vi "DARPA_DoubleJ_20220815_Arduino_ver_newpump.vi"() -> ()   [LabVIEW 2021]
uses:
  <vilib>/Instr/_visa.llb/VISA Configure Serial Port (Instr).vi
  <vilib>/FPGAPlugInAG/PCIe-7857/niLvFpga_Open_PCIe-7857.vi
  <vilib>/rvi/interface/common/dynamic/niFpgaDynamicAddResources.vi
  <vilib>/Utility/error.llb/Error Cluster From Error Code.vi
  <vilib>/rvi/errors/niLvFpgaAdjustHostInterfaceError.vi
  <vilib>/FPGAPlugInAG/Dynamic/niLvFpga_Close_Dynamic.vi
  <vilib>/rvi/interface/nirviOpenFPGA/nirviOpenFPGA.xnode
  FPGA Bitfiles/darpatransitionj_FPGATarget_DARPAFPGADoubleJ_E+A750Kw4Ow.lvbitx
  DARPA_FPGA_DoubleJ_20220715.vi
  <vilib>/rvi/interface/nirviReadWriteControl/nirviReadWriteControl.xnode
  <vilib>/rvi/interface/nirviCloseFPGA/nirviCloseFPGA.xnode
  NiFpgaLv.dll
  <vilib>/rvi/interface/Simulation/niFpgaSimulationCallBeginRW.vi
  <instrlib>/KD Scientific Legato 2XX Series/KD Scientific Legato 2XX Series.lvlib
panel:
  out "Diameter1 (mm)":dbl=4.699
  in  "dia1 (mm)":dbl=0.1 caption="Set Diameter (mm)" min=0.1 max=50.0
  in  "Syringe Selection1":string(combo)="BDP1MM"
  in  "Flow Rate Units (1:ml/min) 2":u32(ring)=1 items=["milliliters per hour (ml/hr)", "milliliters per minute (ml/min)", "milliliters per second (ml/sec)", "microliters per hour (ul/hr)", "microliters per minute (ul/min)", "microliters per second (ul/sec)", "nanoliters per hour (nl/hr)", "nanoliters per minute (nl/min)", "nanoliters per second (nl/sec)", "picoliters per hour (pl/hr)", "picoliters per minute (pl/min)", "picoliters per second (pl/sec)"]
  in  "Flow Rate (5) 2":dbl=5.0 format="%#.4f"
  in  "set param 1":bool
  in  "Baud Rate (115200)":u32(ring)=115200 items=["9600"=9600, "19200"=19200, "38400"=38400, "57600"=57600, "115200"=115200]
  in  "Infuse":bool
  in  "Pause":bool
  in  "Withdraw":bool
  in  "Stop":bool
  out "Infusing":bool
  out "Withdrawing":bool
  out "Idle":bool
  out "Infused Volume":dbl
  out "Withdrawn Volume":dbl
  out "Units (infused)":u16(ring) items=["milliliters", "microliters", "nanoliters", "picoliters"]
  out "Units (withdrawn)":u16(ring) items=["milliliters", "microliters", "nanoliters", "picoliters"]
  in  "VISA resource name":refnum<visa-resource-name>
  out "error out":errorcluster
  in  "stop":bool
  out "Image":u16[][](graph)
  in  "Display":bool=TRUE
  out "Total Frames":i32
  out "Elapsed Time":u32
  out "Software FPS":dbl
  out "Camera FPS":dbl
  in  "H Offset":i32 min=0 max=1604 step=4
  in  "H Width":i32 min=4 max=2304 step=4
  out "SMD":dbl
  out "SHO":i32
  in  "V Offset":i32 min=0 max=1604 step=4
  in  "V Width":i32 min=4 max=2304 step=4
  in  "Binning":u16(ring)=1 items=["1x1"=1, "2x2"=2, "4x4"=4]
  out "SHW":i32
  out "SVO":i32
  out "SVW":i32
  in  "Scan Mode":dbl min=1.0 max=3.0 step=1.0
  in  "Exposure":dbl min=6.576470588235294e-05 max=10.000017235294118 step=1e-08
  out "EXP":dbl
  out "Camera Model":string
  out "Camera Version":string
  out "Camera Serial":string
  in  "Merger on":bool
  in  "ratiocontrol":dbl=1.0
  in  "Arduino COM port":refnum<visa-resource-name>="COM10"
  in  "Arduino \nshut down":bool=TRUE
  in  "Initializer":bool
  out "Serial debugger":string
  in  "PMT2 senstivity":bool
  in  "PMT1 senstivity":bool
  in  "Func amp":bool
  in  "Func Freq":bool
  in  "Func On time":bool
  in  "Func Delay":bool
  in  "PMT1 senstivity input":dbl=0.7 caption="0.5-0.75 V"
  in  "PMT2 senstivity input":dbl caption="0.5-0.75 V"
  in  "Func amp input":dbl=5.0 caption="0 - 5 V"
  in  "Func freq input":dbl=10000.0 caption="100 - 10k Hz"
  in  "Func on Time input":dbl=0.04 caption="0.01 - 1 s"
  in  "Func delay input":dbl caption="0.01 - 1 s"
  out "PMT2 sum":u64(graph)
  out "PMT1 sum":u64(graph)
  out "Unfiltered Signal 1":i16(graph)=643
  out "Filtered Signal 2":i16(graph)=-141
  out "Unfiltered Signal 2":i16(graph)=-138
  in  "Threshold1":dbl=9000.0
  in  "Threshold2":dbl
  out "LabView Timer (sec)":dbl
  out "sample diff":u64
  out "t1 (sample)":u64
  out "t0 (sample)":u64
  out "PMT1 sum":u64
  out "PMT2 sum":u64
  out "Droplet lock on":bool
  out "Filtered Signal1":dbl=373.0
  out "Filtered Signal2":dbl=-141.0
  out "Droplet counter":u64
  out "Unfiltered Signal1":dbl=643.0
  out "Unfiltered Signal2":dbl=-138.0
  in  "Droplet width [ms]":dbl
  in  "determine ratio (xx.xx)":dbl
  out "FPGA loop counter":u64=4737476
  out "Sorted droplet counter":u64
  out "Sort":bool
  in  "FPGA initializer":bool=TRUE
  out "FPGA timer (sec)":dbl=4.737476
  out "FPGA freq":dbl=1000000.0
  out "LabView freq":dbl=8547.008547008547
  out "Filtered Signal 1":i16(graph)=373
  out "PMT1/PMT2":dbl
  out "PMT1/PMT2 (graph)":dbl(graph)
  in  "Output file path":string="D:\\PhD\\00TAMU\\1.research\\nanoBioSystem\\1.projects\\1.DARPA_iSENTRY\\2.src\\LabView\\transition\\FPGA7857_2020\\output files"
  in  "file name":string="tmep"
  out "Confirm path":string="C:\\Data_JJH\\1.Research\\1.projects\\1.DARPA_iSENTRY\\2.src\\LabView\\transition\\FPGA7857_2020\\output files\\20220811 sorting empty 1to500 1.xls"
  out "Data File Ptr":refnum<file>
  # "For inner peace of developers"
  # "Communication Setting"
  # "Sorting Status"
  # "[Pump1] Syringe Setting"
  # "Arduino setting"
  # "PMT display"
  # "Cockpit"
  # "File saving option"
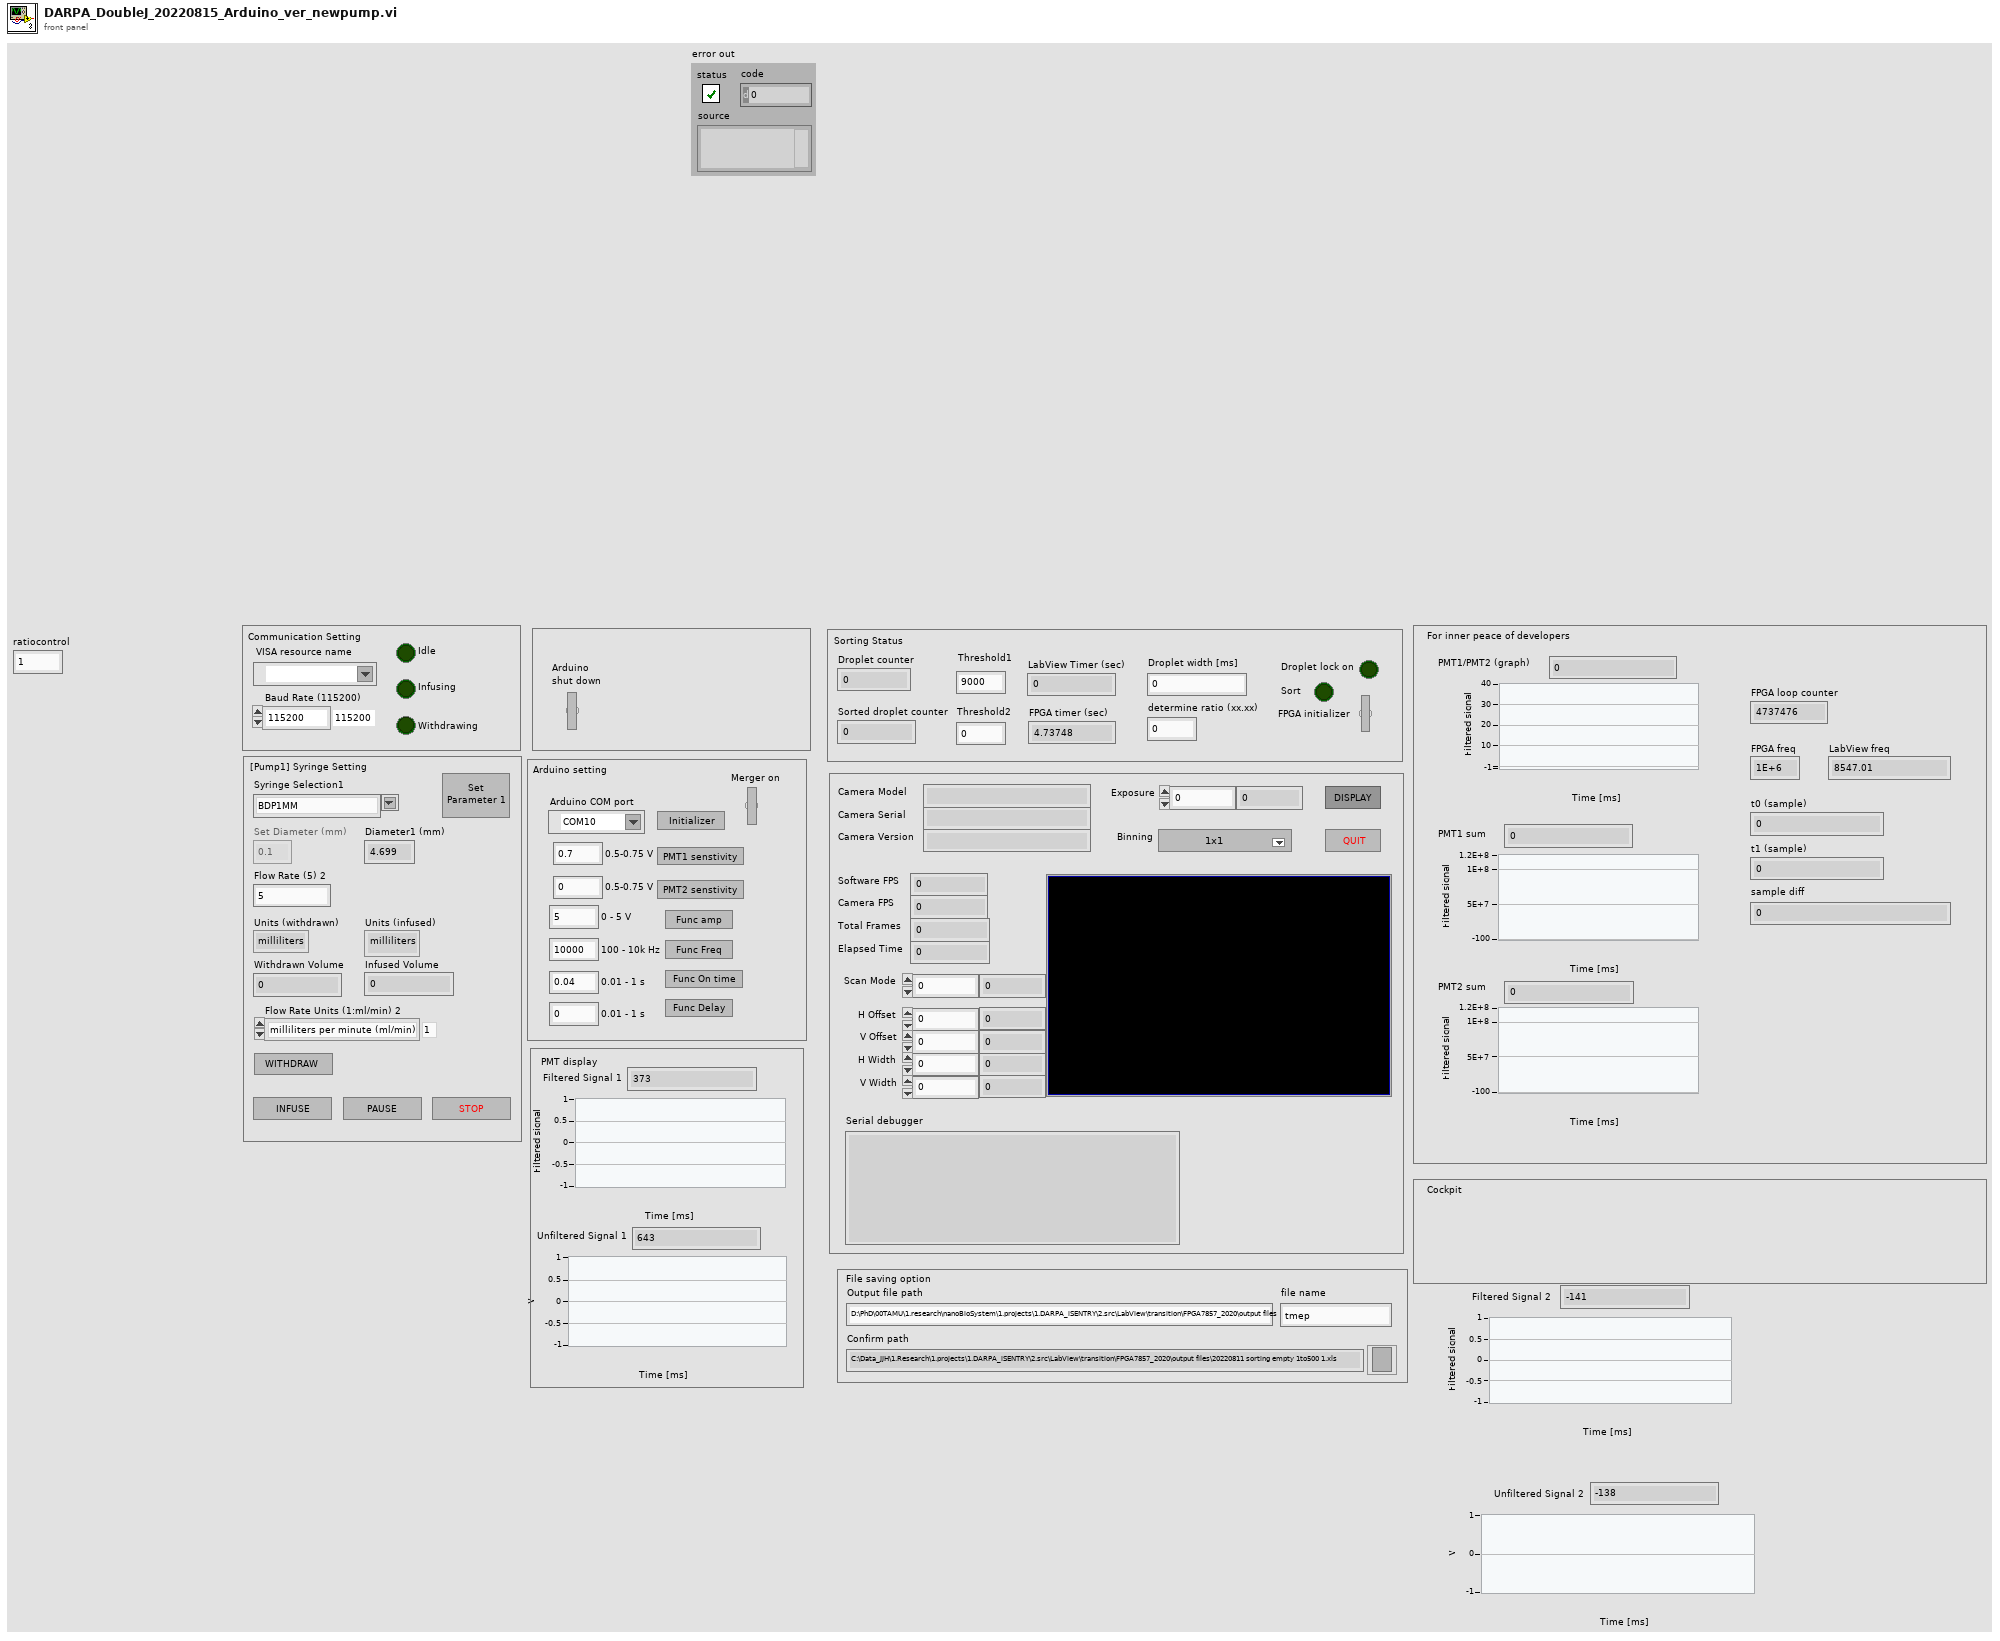
[diagram p1: front panel]
types:
  T1 = enum16{"open", "replace", "create", "open or create", "replace or create", "replace or create with confirmation"}
  T2 = enum8{"Enabled", "Disabled", "Disabled and Grayed Out"}
  T3 = cluster{"Model":string, "Camera ID":string, "Firmware":string}
  T4 = typedef "LVMinMaxIncTypeDef.ctl" = cluster{"Minimum":dbl, "Maximum":dbl, "Increment":dbl}
  T5 = cluster{"H Offset":cluster{"Value":i32, "Limits":T4}, "V Offset":cluster{"Value":i32, "Limits":T4}, "H Size":cluster{"Value":i32, "Limits":T4}, "V Size":cluster{"Value":i32, "Limits":T4}}
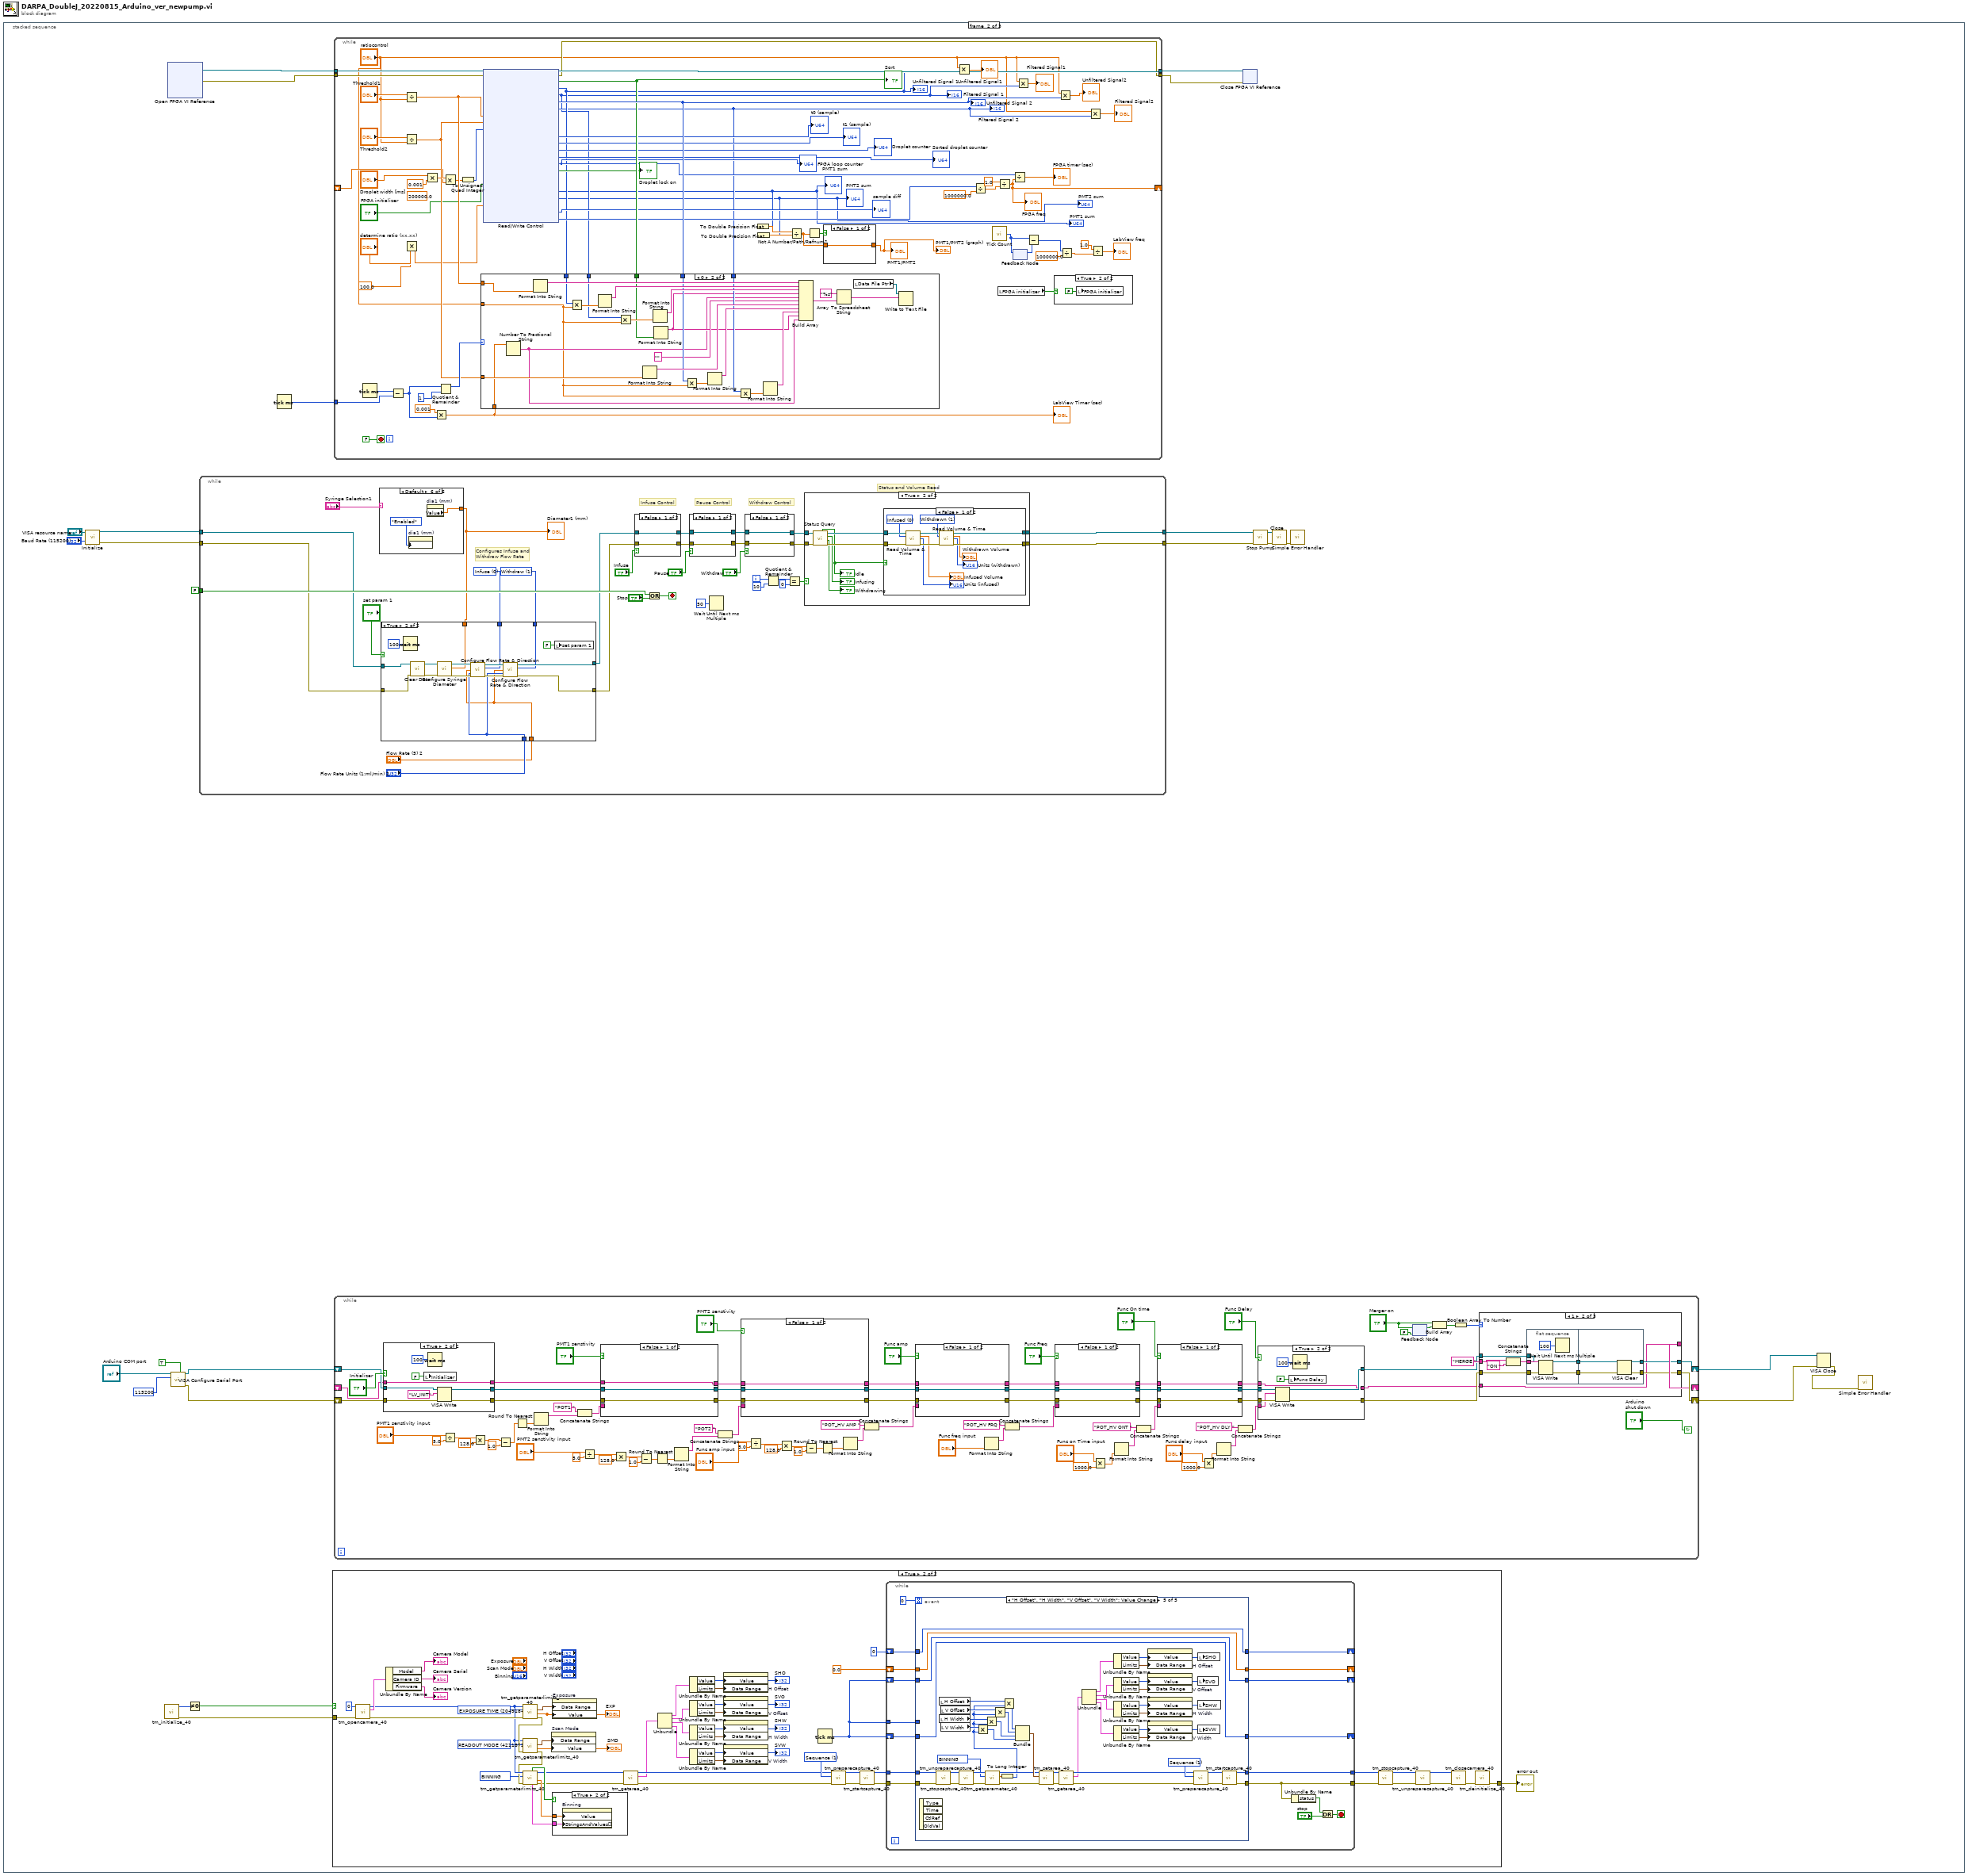
[diagram p0: block diagram]
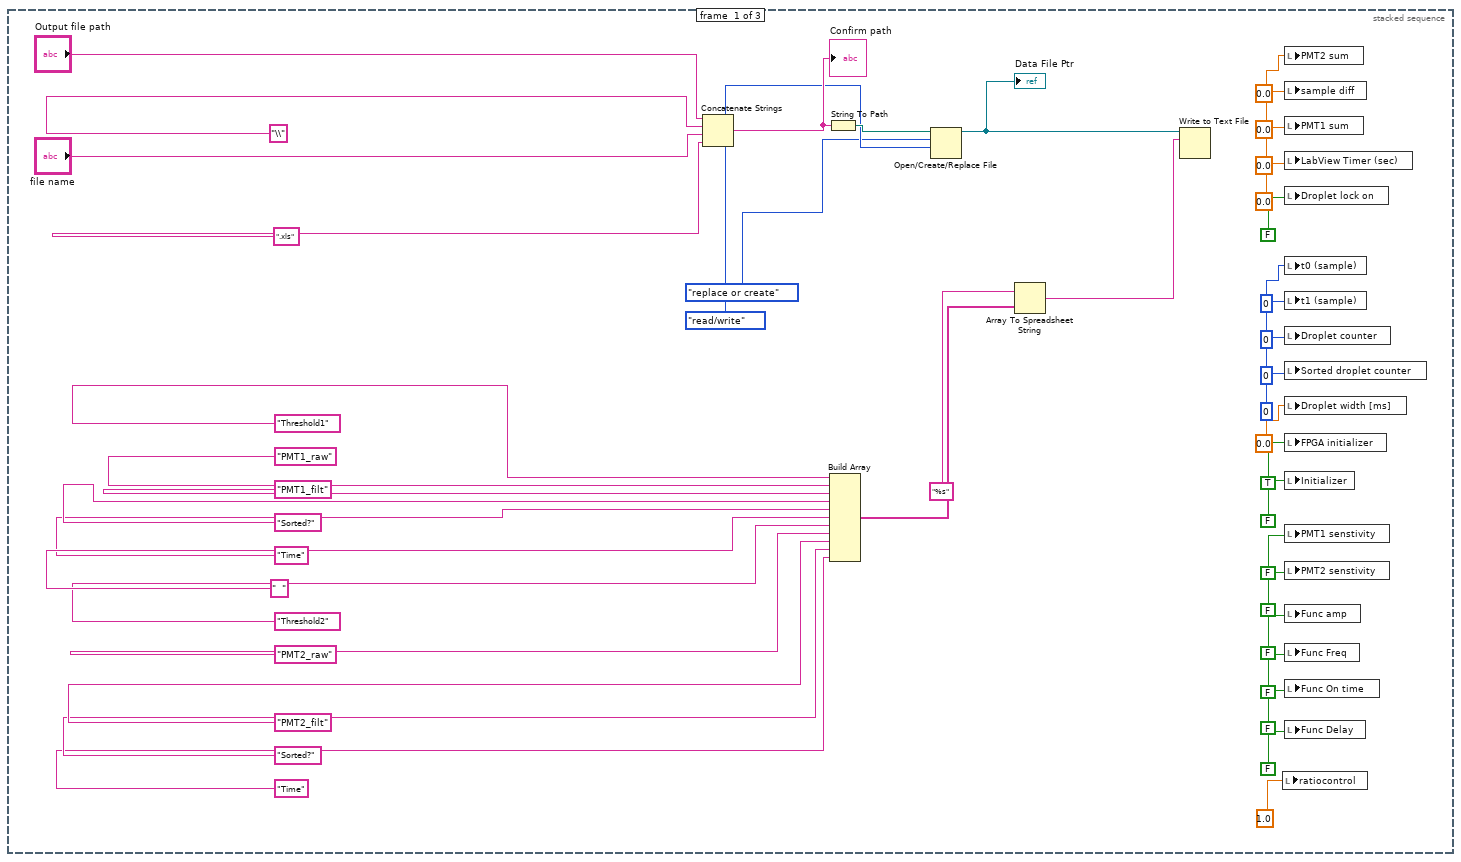
[diagram p2: hidden frame]
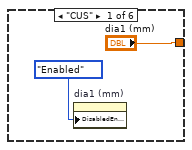
[diagram p3: hidden frame]
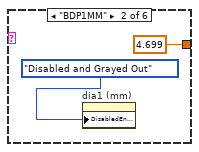
[diagram p4: hidden frame]
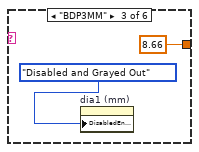
[diagram p5: hidden frame]
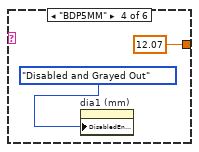
[diagram p6: hidden frame]
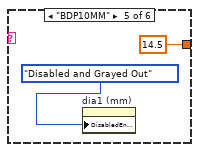
[diagram p7: hidden frame]
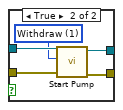
[diagram p11: hidden frame]
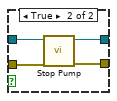
[diagram p12: hidden frame]
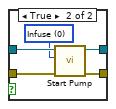
[diagram p13: hidden frame]
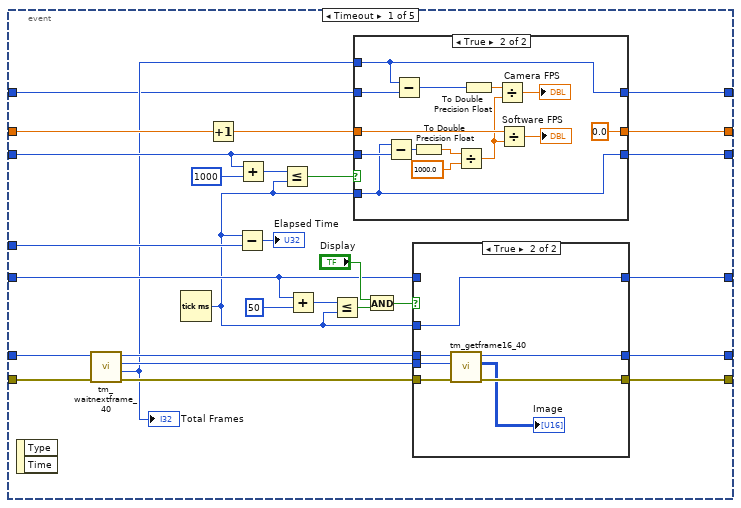
[diagram p16: hidden frame]
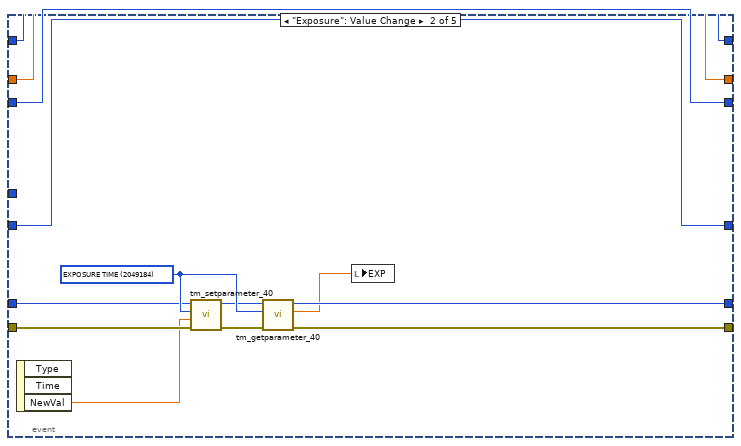
[diagram p19: hidden frame]
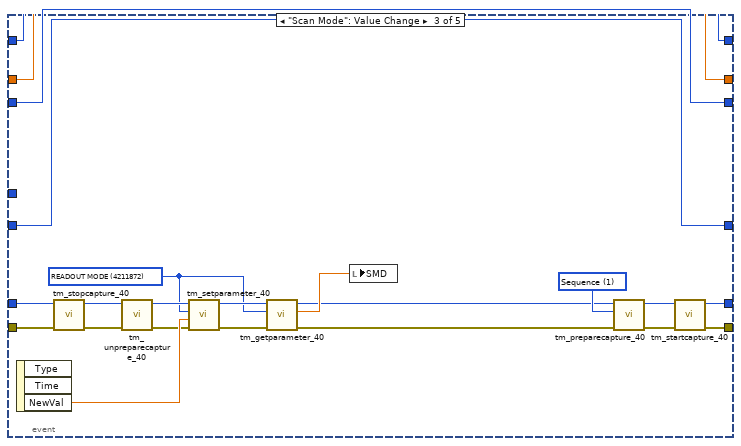
[diagram p20: hidden frame]
diagram:
  n1 = stacked-sequence {
    frame #0 {
      n2 = Concatenate Strings("Output file path", "\\" ("string"), "file name", ".xls" ("string")) -> (w41:string)
      "Confirm path" <- w41
      n3 = String To Path(string=w41) -> (path=w42:path)
      n4 = Build Array("Threshold1", "PMT1_raw", "PMT1_filt", "Sorted?", "Time", "  ", "Threshold2", "PMT2_raw", "PMT2_filt", "Sorted?", "Time") -> (w34:string[])
      n5 = Open/Create/Replace File(file path (use dialog)=w42, operation (0:open)=T1."replace or create", access (0:read/write)=enum16{"read/write", "read-only", "write-only"}."read/write") -> (refnum out=w20:refnum<file>)  [unwired: 3 in, 2 out]
      "Data File Ptr" <- w20
      n6 = Array To Spreadsheet String(array=w34, 3:"%s") -> (spreadsheet string=w22:string)  [unwired: 1 in]
      n7 = Write to Text File(file (use dialog)=w20, text=w22) -> ()  [unwired: 2 in, 3 out]
      n8 = local write "ratiocontrol"(1.0 ("ratiocontrol")) -> ()
      n9 = local write "PMT2 sum"(0.0 ("now")) -> ()
      n10 = local write "sample diff"(0.0 ("sample diff")) -> ()
      n11 = local write "PMT1 sum"(0.0 ("PMT1 sum")) -> ()
      n12 = local write "LabView Timer (sec)"(0.0 ("PMT2 sum")) -> ()
      n13 = local write "Droplet lock on"(FALSE ("Droplet lock on")) -> ()
      n14 = local write "t0 (sample)"(u64 0 ("t0 (sample)")) -> ()
      n15 = local write "t1 (sample)"(u64 0 ("t1 (sample)")) -> ()
      n16 = local write "Droplet counter"(u64 0 ("Droplet counter")) -> ()
      n17 = local write "Sorted droplet counter"(u64 0 ("Sorted droplet counter")) -> ()
      n18 = local write "Droplet width [ms]"(0.0 ("Time compensation [ms]")) -> ()
      n19 = local write "FPGA initializer"(TRUE ("FPGA initializer")) -> ()
      n20 = local write "Initializer"(FALSE ("FPGA initializer")) -> ()
      n21 = local write "PMT1 senstivity"(FALSE ("FPGA initializer")) -> ()
      n22 = local write "PMT2 senstivity"(FALSE ("FPGA initializer")) -> ()
      n23 = local write "Func amp"(FALSE ("FPGA initializer")) -> ()
      n24 = local write "Func Freq"(FALSE ("FPGA initializer")) -> ()
      n25 = local write "Func On time"(FALSE ("FPGA initializer")) -> ()
      n26 = local write "Func Delay"(FALSE ("FPGA initializer")) -> ()
    }
    frame #1 {
      n27 = call <instrlib>:"Initialize.vi"("Baud Rate (115200)"="Baud Rate (115200)", "VISA resource name"="VISA resource name") -> ("error out"=w44:errorcluster, "VISA resource name out"=w45:refnum<visa-resource-name>)  [unwired: 8 in]
      n28 = call <userlib>:"tm_initialize_40.vi"() -> ("error out"=w54:errorcluster, "Number Of Cameras"=w53:u32)  [unwired: 8 in, 2 out]
      n29 = xnode "Open FPGA VI Reference"() -> ("FPGA VI Reference Out"=w69:refnum<k20>, "error out"=w68:errorcluster)  [unwired: 2 in]
      n30 = call-poly "VISA Configure Serial Port"("VISA resource name"="Arduino COM port", "Enable Termination\nChar (T)"=TRUE ("Enable Termination\nChar (T)"), "baud rate (9600)"=u32 115200) -> ("VISA resource name out"=w60:refnum<visa-resource-name>, "error out"=w59:errorcluster)  [unwired: 11 in]
      n31 = Not Equal To 0?(x=w53) -> (x != 0?=w56:bool)
      n32 = while {
        tunnel: w45 -> [w79]
        tunnel: w44 -> [w77]
        tunnel: [w91] -> w48
        tunnel: [w90] -> w47
        tunnel: FALSE -> [w82]
        i -> [w88]
        stop <- w84 stop-if-true
        w73 = u16 0 items=["Infuse", "Withdraw"] ("Pump Method (0:Infuse)")
        w72 = u16 1 items=["Infuse", "Withdraw"] ("Pump Method (0:Infuse)")
        # "Configures Infuse and Withdraw Flow Rate"
        # "Withdraw Control"
        # "Pause Control"
        # "Infuse Control"
        # "Status and Volume Read"
        n33 = case shown="Default" "Syringe Selection1" {
          tunnel: ["dia1 (mm)" 4.699 ("dia (mm)") 8.66 ("dia (mm)") 12.07 ("dia (mm)") 14.5 ("dia (mm)") w112] -> w70
          frame "CUS" {
            n34 = property on="dia1 (mm)" class="DigNum (strict)"("DisabledEnum"=T2."Enabled" ("Disabled")) -> ()  [unwired: 2 in, 2 out]
          }
          frame "BDP1MM" {
            n35 = property on="dia1 (mm)" class="DigNum (strict)"("DisabledEnum"=T2."Disabled and Grayed Out" ("Disabled")) -> ()  [unwired: 2 in, 2 out]
          }
          frame "BDP3MM" {
            n36 = property on="dia1 (mm)" class="DigNum (strict)"("DisabledEnum"=T2."Disabled and Grayed Out" ("Disabled")) -> ()  [unwired: 2 in, 2 out]
          }
          frame "BDP5MM" {
            n37 = property on="dia1 (mm)" class="DigNum (strict)"("DisabledEnum"=T2."Disabled and Grayed Out" ("Disabled")) -> ()  [unwired: 2 in, 2 out]
          }
          frame "BDP10MM" {
            n38 = property on="dia1 (mm)" class="DigNum (strict)"("DisabledEnum"=T2."Disabled and Grayed Out" ("Disabled")) -> ()  [unwired: 2 in, 2 out]
          }
          frame Default {
            n39 = property on="dia1 (mm)" class="DigNum (strict)"("DisabledEnum"=T2."Enabled" ("Disabled")) -> ()  [unwired: 2 in, 2 out]
            n40 = property on="dia1 (mm)" class="DigNum (strict)"() -> ("Value"=w112:dbl)  [unwired: 2 in, 2 out]
          }
        }
        "Diameter1 (mm)" <- w70
        n41 = case shown="True" "set param 1" {
          tunnel: w79 -> [w114 w125]
          tunnel: [w114 w123] -> w78
          tunnel: w77 -> [w113 w124]
          tunnel: [w113 w122] -> w76
          tunnel: "Flow Rate Units (1:ml/min) 2" -> [_ w121]
          tunnel: "Flow Rate (5) 2" -> [_ w120]
          tunnel: w70 -> [_ w119]
          tunnel: w73 -> [_ w118]
          tunnel: w72 -> [_ w117]
          frame False {
          }
          frame True {
            n42 = Wait (ms)(milliseconds to wait=u32 100) -> ()  [unwired: 1 out]
            n43 = call <instrlib>:"Clear Data.vi"("error in (no error)"=w124, "VISA resource name"=w125) -> ("error out"=w130:errorcluster, "VISA resource name out"=w131:refnum<visa-resource-name>)  [unwired: 8 in]
            n44 = call <instrlib>:"Configure Syringe Diameter.vi"("error in (no error)"=w130, "Syringe Diameter (20 mm)"=w119, "VISA resource name"=w131) -> ("error out"=w127:errorcluster, "VISA resource name out"=w128:refnum<visa-resource-name>)  [unwired: 7 in]
            n45 = call <instrlib>:"Configure Flow Rate & Direction.vi"("VISA resource name"=w128, "Pump Direction (0:Infuse)"=w118, "Flow Rate (5.00)"=w120, "Flow Rate Units (1:ml/min)"=w121, "error in (no error)"=w127) -> ("VISA resource name out"=w129:refnum<visa-resource-name>, "error out"=w126:errorcluster)  [unwired: 9 in]
            n46 = call <instrlib>:"Configure Flow Rate & Direction.vi"("VISA resource name"=w129, "Pump Direction (0:Infuse)"=w117, "Flow Rate (5.00)"=w120, "Flow Rate Units (1:ml/min)"=w121, "error in (no error)"=w126) -> ("VISA resource name out"=w123:refnum<visa-resource-name>, "error out"=w122:errorcluster)  [unwired: 9 in]
            n47 = local write "set param 1"(FALSE ("set param 1")) -> ()
          }
        }
        n48 = case shown="False" "Infuse" {
          tunnel: w78 -> [w171 w176]
          tunnel: w76 -> [w170 w175]
          tunnel: [w171 w174] -> w98
          tunnel: [w170 w173] -> w97
          frame False {
          }
          frame True {
            w172 = u16 0 items=["Infuse", "Withdraw"] ("Run Method (0:Infuse)")
            n49 = call <instrlib>:"Start Pump.vi"("error in (no error)"=w175, "Run Direction (0:Infuse)"=w172, "VISA resource name"=w176) -> ("error out"=w173:errorcluster, "VISA resource name out"=w174:refnum<visa-resource-name>)  [unwired: 7 in]
          }
        }
        n50 = Or(x=w82, y="Stop") -> (x .or. y?=w84:bool)
        n51 = case shown="False" "Pause" {
          tunnel: w98 -> [w165 w169]
          tunnel: w97 -> [w164 w168]
          tunnel: [w165 w167] -> w96
          tunnel: [w164 w166] -> w95
          frame False {
          }
          frame True {
            n52 = call <instrlib>:"Stop Pump.vi"("error in (no error)"=w168, "VISA resource name"=w169) -> ("error out"=w166:errorcluster, "VISA resource name out"=w167:refnum<visa-resource-name>)  [unwired: 8 in]
          }
        }
        n53 = Wait Until Next ms Multiple(millisecond multiple=u32 50) -> ()  [unwired: 1 out]
        n54 = case shown="False" "Withdraw" {
          tunnel: w96 -> [w158 w163]
          tunnel: w95 -> [w157 w162]
          tunnel: [w158 w161] -> w93
          tunnel: [w157 w160] -> w92
          frame False {
          }
          frame True {
            w159 = u16 1 items=["Infuse", "Withdraw"] ("Run Method (0:Infuse)")
            n55 = call <instrlib>:"Start Pump.vi"("error in (no error)"=w162, "Run Direction (0:Infuse)"=w159, "VISA resource name"=w163) -> ("error out"=w160:errorcluster, "VISA resource name out"=w161:refnum<visa-resource-name>)  [unwired: 7 in]
          }
        }
        n56 = Quotient & Remainder(x=w88, y=10) -> (x-y*floor(x/y)=w86:i32)  [unwired: 1 out]
        n57 = Equal?(x=w86, y=0) -> (x = y?=w81:bool)
        n58 = case shown="True" w81 {
          tunnel: w93 -> [w133 w138]
          tunnel: w92 -> [w132 w137]
          tunnel: [w133 w136] -> w91
          tunnel: [w132 w135] -> w90
          frame False {
            # "Reads Status and Volume once every 10 iteration of the while loop to prevent the instrument from receiving too many commands."
          }
          frame True {
            n59 = call <instrlib>:"Status Query.vi"("error in (no error)"=w137, "VISA resource name"=w138) -> ("error out"=w142:errorcluster, "Withdrawing"=→"Withdrawing":bool, "Infusing"=→"Infusing":bool, "VISA resource name out"=w141:refnum<visa-resource-name>, "Idle"=w134:bool)  [unwired: 4 in, 1 out]
            "Idle" <- w134
            n60 = case shown="False" w134 {
              tunnel: w142 -> [w154 w155]
              tunnel: w141 -> [w153 w156]
              tunnel: [w152 w156] -> w136
              tunnel: [w151 w155] -> w135
              frame False {
                w147 = u16 0 items=["Infused", "Withdrawn"] ("Pump Method (0:Infused)")
                w148 = u16 1 items=["Infused", "Withdrawn"] ("Pump Method (0:Infused)")
                n61 = call <instrlib>:"Read Volume & Time .vi"("VISA resource name"=w153, "Pump Direction (0:Infused)"=w147, "error in (no error)"=w154) -> ("VISA resource name out"=w149:refnum<visa-resource-name>, "Volume"=→"Infused Volume":dbl, "Volume Units"=→"Units (infused)":u16, "error out"=w150:errorcluster)  [unwired: 7 in, 2 out]
                n62 = call <instrlib>:"Read Volume & Time .vi"("VISA resource name"=w149, "Pump Direction (0:Infused)"=w148, "error in (no error)"=w150) -> ("VISA resource name out"=w152:refnum<visa-resource-name>, "Volume"=→"Withdrawn Volume":dbl, "Volume Units"=→"Units (withdrawn)":u16, "error out"=w151:errorcluster)  [unwired: 7 in, 2 out]
              }
              frame True {
                # "Reads Volume only when the pump is infusing or withdrawing. This will reduce the commands sent to the instrument and prevents the instrument having errors."
              }
            }
          }
        }
      }
      n63 = Tick Count (ms)() -> (millisecond timer value=w65:u32)
      n64 = case shown="True" w56 {
        tunnel: [w177 w227] -> w55
        tunnel: w54 -> [w177 w230]
        frame False {
        }
        frame True {
          w199 = u32 2049184 items=["BINNING"=4215968, "BITS PER CHANNEL"=4342976, "ACTIVE VIEW INDEX"=4343136, "CCD MODE"=4212384, "SENSOR MODE"=4212128, "READOUT MODE"=4211872, "EXPOSURE TIME"=2049184, "CONTRAST GAIN"=3163312, "CONTRAST OFFSET"=3163328, "LIGHT MODE"=2114720, "SENSITIVITY"=2114992, "WHITE BALANCE"=3163568, "PHOTON IMAGING MODE"=2115200, "HIGH DYNAMIC RANGE MODE"=3163360, "TRIGGER SOURCE"=1066144, "TRIGGER ACTIVE"=1066160, "TRIGGER MODE"=1066400, "TRIGGER POLARITY"=1066416, "TRIGGER GLOBAL EXPOSURE"=2049680, "FIRST TRIGGER BEHAVIOR"=2049696, "TRIGGER TIMES"=1066448, "OUTPUT TRIGGER POLARITY"=1852592, "OUTPUT TRIGGER DELAY"=1852624, "OUTPUT TRIGGER PERIOD"=1852640, "TEMPERATURE"=2115232, "TEMPERATURE TARGET"=2115264, "SENSOR COOLER FAN"=2115296, "MECHANICAL SHUTTER"=2115488, "BACK FOCUS POSITION"=8422304, "FRAMEBUNDLE MODE"=4346784, "FRAMEBUNDLE NUMBER"=4346800, "LINEBUNDLE HEIGHT"=4212192, "TRIGGER CONNECTOR"=1066432, "IMAGE PIXEL TYPE"=4343296, "OUTPUT TRIGGER KIND"=1852656, "READOUT DIRECTION"=4211904, "CHANNEL SYNC"=1852352] ("Parameter")
          w200 = u32 4211872 items=["BINNING"=4215968, "BITS PER CHANNEL"=4342976, "ACTIVE VIEW INDEX"=4343136, "CCD MODE"=4212384, "SENSOR MODE"=4212128, "READOUT MODE"=4211872, "EXPOSURE TIME"=2049184, "CONTRAST GAIN"=3163312, "CONTRAST OFFSET"=3163328, "LIGHT MODE"=2114720, "SENSITIVITY"=2114992, "WHITE BALANCE"=3163568, "PHOTON IMAGING MODE"=2115200, "HIGH DYNAMIC RANGE MODE"=3163360, "TRIGGER SOURCE"=1066144, "TRIGGER ACTIVE"=1066160, "TRIGGER MODE"=1066400, "TRIGGER POLARITY"=1066416, "TRIGGER GLOBAL EXPOSURE"=2049680, "FIRST TRIGGER BEHAVIOR"=2049696, "TRIGGER TIMES"=1066448, "OUTPUT TRIGGER POLARITY"=1852592, "OUTPUT TRIGGER DELAY"=1852624, "OUTPUT TRIGGER PERIOD"=1852640, "TEMPERATURE"=2115232, "TEMPERATURE TARGET"=2115264, "SENSOR COOLER FAN"=2115296, "MECHANICAL SHUTTER"=2115488, "BACK FOCUS POSITION"=8422304, "FRAMEBUNDLE MODE"=4346784, "FRAMEBUNDLE NUMBER"=4346800, "LINEBUNDLE HEIGHT"=4212192, "TRIGGER CONNECTOR"=1066432, "IMAGE PIXEL TYPE"=4343296, "OUTPUT TRIGGER KIND"=1852656, "READOUT DIRECTION"=4211904, "CHANNEL SYNC"=1852352] ("Parameter")
          w201 = u32 4215968 items=["BINNING"=4215968, "BITS PER CHANNEL"=4342976, "ACTIVE VIEW INDEX"=4343136, "CCD MODE"=4212384, "SENSOR MODE"=4212128, "READOUT MODE"=4211872, "EXPOSURE TIME"=2049184, "CONTRAST GAIN"=3163312, "CONTRAST OFFSET"=3163328, "LIGHT MODE"=2114720, "SENSITIVITY"=2114992, "WHITE BALANCE"=3163568, "PHOTON IMAGING MODE"=2115200, "HIGH DYNAMIC RANGE MODE"=3163360, "TRIGGER SOURCE"=1066144, "TRIGGER ACTIVE"=1066160, "TRIGGER MODE"=1066400, "TRIGGER POLARITY"=1066416, "TRIGGER GLOBAL EXPOSURE"=2049680, "FIRST TRIGGER BEHAVIOR"=2049696, "TRIGGER TIMES"=1066448, "OUTPUT TRIGGER POLARITY"=1852592, "OUTPUT TRIGGER DELAY"=1852624, "OUTPUT TRIGGER PERIOD"=1852640, "TEMPERATURE"=2115232, "TEMPERATURE TARGET"=2115264, "SENSOR COOLER FAN"=2115296, "MECHANICAL SHUTTER"=2115488, "BACK FOCUS POSITION"=8422304, "FRAMEBUNDLE MODE"=4346784, "FRAMEBUNDLE NUMBER"=4346800, "LINEBUNDLE HEIGHT"=4212192, "TRIGGER CONNECTOR"=1066432, "IMAGE PIXEL TYPE"=4343296, "OUTPUT TRIGGER KIND"=1852656, "READOUT DIRECTION"=4211904, "CHANNEL SYNC"=1852352] ("Parameter")
          w225 = 1 items=["Snap", "Sequence"] ("Capture mode")
          n65 = call <userlib>:"tm_opencamera_40.vi"("error in (no error)"=w230, "Camera Index"=u32 0) -> ("error out"=w208:errorcluster, "Camera Details"=w212:T3, "Handle out"=w206:u32)  [unwired: 7 in]
          n66 = Unbundle By Name(w212) -> ("Model"=→"Camera Model":string, "Camera ID"=→"Camera Serial":string, "Firmware"=→"Camera Version":string)
          n67 = call <userlib>:"tm_getparameterlimits_40.vi"("error in (no error)"=w208, "Parameter"=w199, "Handle in"=w206) -> ("error out"=w207:errorcluster, "default"=w191:dbl, "Range"=w192:cluster{"min":dbl, "max":dbl, "step":dbl})  [unwired: 2 in, 4 out]
          "EXP" <- w191
          n68 = call <userlib>:"tm_getparameterlimits_40.vi"("error in (no error)"=w207, "Parameter"=w200, "Handle in"=w206) -> ("error out"=w205:errorcluster, "default"=w193:dbl, "Range"=w194:cluster{"min":dbl, "max":dbl, "step":dbl})  [unwired: 2 in, 4 out]
          "SMD" <- w193
          n69 = call <userlib>:"tm_getparameterlimits_40.vi"("error in (no error)"=w205, "Parameter"=w201, "Handle in"=w206) -> ("error out"=w198:errorcluster, "default"=w203:dbl, "Handle out"=w197:u32, "Value Names"=w202:cluster{"Name":string, "Value":dbl}[], "Writable"=w204:bool)  [unwired: 2 in, 2 out]
          n70 = property on="Scan Mode" class="DigNum (strict)"("Data Range"=w194, "Value"=w193) -> ()  [unwired: 2 in, 2 out]
          n71 = property on="Exposure" class="DigNum (strict)"("Data Range"=w192, "Value"=w191) -> ()  [unwired: 2 in, 2 out]
          n72 = case shown="True" w204 {
            tunnel: w202 -> [_ w232]
            tunnel: w203 -> [_ w231]
            frame False {
            }
            frame True {
              n73 = property on="Binning" class="Ring (strict)"("Value"=w231, "StringsAndValues[]"=w232) -> ()  [unwired: 2 in, 2 out]
            }
          }
          n74 = call <userlib>:"tm_getarea_40.vi"("error in (no error)"=w198, "Handle in"=w197) -> ("error out"=w196:errorcluster, "Sub Region"=w186:T5, "Handle out"=w195:u32)  [unwired: 7 in]
          n75 = Unbundle(w186) -> ("H Offset"=w190:cluster{"Value":i32, "Limits":T4}, "V Offset"=w189:cluster{"Value":i32, "Limits":T4}, "H Size"=w188:cluster{"Value":i32, "Limits":T4}, "V Size"=w187:cluster{"Value":i32, "Limits":T4})
          n76 = Unbundle By Name(w190) -> ("Value"=w185:i32, "Limits"=w184:T4)
          "SHO" <- w185
          n77 = Unbundle By Name(w189) -> ("Value"=w179:i32, "Limits"=w178:T4)
          "SVO" <- w179
          n78 = Unbundle By Name(w188) -> ("Value"=w181:i32, "Limits"=w180:T4)
          "SHW" <- w181
          n79 = Unbundle By Name(w187) -> ("Value"=w183:i32, "Limits"=w182:T4)
          "SVW" <- w183
          n80 = property on="H Offset" class="DigNum (strict)"("Value"=w185, "Data Range"=w184) -> ()  [unwired: 2 in, 2 out]
          n81 = property on="V Offset" class="DigNum (strict)"("Value"=w179, "Data Range"=w178) -> ()  [unwired: 2 in, 2 out]
          n82 = property on="H Width" class="DigNum (strict)"("Value"=w181, "Data Range"=w180) -> ()  [unwired: 2 in, 2 out]
          n83 = property on="V Width" class="DigNum (strict)"("Value"=w183, "Data Range"=w182) -> ()  [unwired: 2 in, 2 out]
          n84 = Tick Count (ms)() -> (millisecond timer value=w220:u32)
          n85 = call <userlib>:"tm_preparecapture_40.vi"("error in (no error)"=w196, "Capture mode"=w225, "Handle in"=w195) -> ("error out"=w223:errorcluster, "Handle out"=w224:u32)  [unwired: 5 in, 2 out]
          n86 = call <userlib>:"tm_startcapture_40.vi"("error in (no error)"=w223, "Handle in"=w224) -> ("error out"=w222:errorcluster, "Handle out"=w221:u32)  [unwired: 8 in]
          n87 = while {
            tunnel: w222 -> [w239]
            tunnel: [w237] -> w219
            tunnel: [w236] -> w218
            shift-right: [w245] -> _
            shift-left: w220 -> [w243]
            shift-right: [w246] -> _
            shift-left: 0.0 -> [w244]
            shift-right: [w238] -> _
            shift-left: w220 -> [w241]
            tunnel: w221 -> [w240]
            tunnel: w220 -> [w242]
            shift-right: [w233] -> _
            shift-left: 0 -> [w234]
            stop <- w247 stop-if-true
            n88 = event shown="[4] \"H Offset\", \"H Width\", \"V Offset\", \"V Width\": Value Change" {
              selector: _ -> [_ _ _ _ _]
              dyn-events: _ -> [_ _ _ _ _]
              timeout: 0 -> [_ _ _ _ _]
              tunnel: [w254 w315 w337 w366 w412] -> w246
              tunnel: [w253 w316 w338 w367 w413] -> w245
              tunnel: w244 -> [w263 w315 w337 w366 w412]
              tunnel: w243 -> [w256 w316 w338 w367 w413]
              tunnel: w242 -> [w259 _ _ _ _]
              tunnel: w241 -> [w264 w317 w339 w373 w419]
              tunnel: w240 -> [w266 w310 w334 w365 w410]
              tunnel: w239 -> [w265 w312 w333 w364 w409]
              tunnel: [w262 w317 w339 w373 w419] -> w238
              tunnel: [w261 w307 w328 w368 w414] -> w237
              tunnel: [w260 w305 w329 w369 w415] -> w236
              tunnel: w234 -> [w251 w314 w327 w361 w406]
              tunnel: [w250 w314 w327 w361 w406] -> w233
              event Timeout {
                n89 = event-data() -> ()  [unwired: 1 in, 2 out]
                n90 = call <userlib>:"tm_waitnextframe_40.vi"("error in (no error)"=w265, "Handle in"=w266) -> ("error out"=w270:errorcluster, "Frame Count"=w252:i32, "Frame Index"=w269:i32, "Handle out"=w271:u32)  [unwired: 6 in]
                "Total Frames" <- w252
                n91 = Tick Count (ms)() -> (millisecond timer value=w258:u32)
                n92 = Increment(x=w263) -> (x+1=w255:dbl)
                n93 = Subtract(x=w258, y=w259) -> (x-y=→"Elapsed Time":u32)
                n94 = Add(x=w256, y=u32 1000) -> (x+y=w277:u32)
                n95 = Less Or Equal?(x=w277, y=w258) -> (x <= y?=w257:bool)
                n96 = Add(x=w264, y=u32 50) -> (x+y=w275:u32)
                n97 = Less Or Equal?(x=w275, y=w258) -> (x <= y?=w273:bool)
                n98 = case shown="True" w257 {
                  tunnel: w256 -> [w280 w289]
                  tunnel: [w280 w286] -> w253
                  tunnel: w255 -> [w279 w292]
                  tunnel: w258 -> [_ w286]
                  tunnel: [w279 0.0] -> w254
                  tunnel: w252 -> [_ w281]
                  tunnel: w251 -> [w278 w284]
                  tunnel: [w278 w281] -> w250
                  frame False {
                  }
                  frame True {
                    n99 = Subtract(x=w286, y=w289) -> (x-y=w288:u32)
                    n100 = Subtract(x=w281, y=w284) -> (x-y=w282:i32)
                    n101 = To Double Precision Float(number=w288) -> (double precision float=w294:dbl)
                    n102 = Divide(x=w294, y=1000.0) -> (x/y=w285:dbl)
                    n103 = To Double Precision Float(number=w282) -> (double precision float=w283:dbl)
                    n104 = Divide(x=w283, y=w285) -> (x/y=→"Camera FPS":dbl)
                    n105 = Divide(x=w292, y=w285) -> (x/y=→"Software FPS":dbl)
                  }
                }
                n106 = And(x="Display", y=w273) -> (x .and. y?=w268:bool)
                n107 = case shown="True" w268 {
                  tunnel: w264 -> [w297 _]
                  tunnel: w258 -> [_ w304]
                  tunnel: [w297 w304] -> w262
                  tunnel: w271 -> [w296 w303]
                  tunnel: w270 -> [w295 w302]
                  tunnel: [w296 w301] -> w261
                  tunnel: [w295 w300] -> w260
                  tunnel: w269 -> [_ w298]
                  frame False {
                  }
                  frame True {
                    n108 = call <userlib>:"tm_getframe16_40.vi"("error in (no error)"=w302, "Frame Index"=w298, "Handle in"=w303) -> ("error out"=w300:errorcluster, "Data"=→"Image":u16[][], "Handle out"=w301:u32)  [unwired: 5 in, 1 out]
                  }
                }
              }
              event "Exposure": Value Change {
                w313 = u32 2049184 items=["SENSOR MODE"=4212128, "CCD MODE"=4212384, "READOUT MODE"=4211872, "ACTIVE VIEW INDEX"=4343136, "BITS PER CHANNEL"=4342976, "IMAGE PIXEL TYPE"=4343296, "BINNING"=4215968, "EXPOSURE TIME"=2049184, "CONTRAST GAIN"=3163312, "CONTRAST OFFSET"=3163328, "LIGHT MODE"=2114720, "SENSITIVITY"=2114992, "PHOTON IMAGING MODE"=2115200, "HIGH DYNAMIC RANGE MODE"=3163360, "WHITE BALANCE"=3163568, "TEMPERATURE"=2115232, "TEMPERATURE TARGET"=2115264, "SENSOR COOLER FAN"=2115296, "LINEBUNDLE HEIGHT"=4212192, "MECHANICAL SHUTTER"=2115488, "BACK FOCUS POSITION"=8422304, "TRIGGER CONNECTOR"=1066432, "TRIGGER SOURCE"=1066144, "OUTPUT TRIGGER SOURCE"=1852576, "TRIGGER GLOBAL EXPOSURE"=2049680, "FIRST TRIGGER BEHAVIOR"=2049696, "CHANNEL SYNC"=1852352, "READOUT DIRECTION"=4211904, "PRE HSYNC COUNT"=1852704] ("Parameter")
                n109 = event-data() -> ("NewVal"=w311:dbl)  [unwired: 1 in, 2 out]
                n110 = call <userlib>:"tm_setparameter_40.vi"("error in (no error)"=w312, "Value in"=w311, "Parameter"=w313, "Handle in"=w310) -> ("error out"=w309:errorcluster, "Handle out"=w308:u32)  [unwired: 6 in]
                n111 = call <userlib>:"tm_getparameter_40.vi"("error in (no error)"=w309, "Parameter"=w313, "Handle in"=w308) -> ("error out"=w305:errorcluster, "Value out"=w306:dbl, "Handle out"=w307:u32)  [unwired: 6 in]
                n112 = local write "EXP"(w306) -> ()
              }
              event "Scan Mode": Value Change {
                w318 = u32 4211872 items=["SENSOR MODE"=4212128, "CCD MODE"=4212384, "READOUT MODE"=4211872, "ACTIVE VIEW INDEX"=4343136, "BITS PER CHANNEL"=4342976, "IMAGE PIXEL TYPE"=4343296, "BINNING"=4215968, "EXPOSURE TIME"=2049184, "CONTRAST GAIN"=3163312, "CONTRAST OFFSET"=3163328, "LIGHT MODE"=2114720, "SENSITIVITY"=2114992, "PHOTON IMAGING MODE"=2115200, "HIGH DYNAMIC RANGE MODE"=3163360, "WHITE BALANCE"=3163568, "TEMPERATURE"=2115232, "TEMPERATURE TARGET"=2115264, "SENSOR COOLER FAN"=2115296, "LINEBUNDLE HEIGHT"=4212192, "MECHANICAL SHUTTER"=2115488, "BACK FOCUS POSITION"=8422304, "TRIGGER CONNECTOR"=1066432, "TRIGGER SOURCE"=1066144, "OUTPUT TRIGGER SOURCE"=1852576, "TRIGGER GLOBAL EXPOSURE"=2049680, "FIRST TRIGGER BEHAVIOR"=2049696, "CHANNEL SYNC"=1852352, "READOUT DIRECTION"=4211904, "PRE HSYNC COUNT"=1852704] ("Parameter")
                w332 = 1 items=["Snap", "Sequence"] ("Capture mode")
                n113 = event-data() -> ("NewVal"=w323:dbl)  [unwired: 1 in, 2 out]
                n114 = call <userlib>:"tm_stopcapture_40.vi"("error in (no error)"=w333, "Handle in"=w334) -> ("error out"=w335:errorcluster, "Handle out"=w336:u32)  [unwired: 8 in]
                n115 = call <userlib>:"tm_unpreparecapture_40.vi"("error in (no error)"=w335, "Handle in"=w336) -> ("error out"=w321:errorcluster, "Handle out"=w322:u32)  [unwired: 8 in]
                n116 = call <userlib>:"tm_setparameter_40.vi"("error in (no error)"=w321, "Value in"=w323, "Parameter"=w318, "Handle in"=w322) -> ("error out"=w320:errorcluster, "Handle out"=w319:u32)  [unwired: 6 in]
                n117 = call <userlib>:"tm_getparameter_40.vi"("error in (no error)"=w320, "Parameter"=w318, "Handle in"=w319) -> ("error out"=w326:errorcluster, "Value out"=w325:dbl, "Handle out"=w324:u32)  [unwired: 6 in]
                n118 = local write "SMD"(w325) -> ()
                n119 = call <userlib>:"tm_preparecapture_40.vi"("error in (no error)"=w326, "Capture mode"=w332, "Handle in"=w324) -> ("error out"=w330:errorcluster, "Handle out"=w331:u32)  [unwired: 5 in, 2 out]
                n120 = call <userlib>:"tm_startcapture_40.vi"("error in (no error)"=w330, "Handle in"=w331) -> ("error out"=w329:errorcluster, "Handle out"=w328:u32)  [unwired: 8 in]
              }
              event "Binning": Value Change {
                w359 = u32 4215968 items=["BINNING"=4215968, "BITS PER CHANNEL"=2, "ACTIVE VIEW INDEX"=3, "CCD MODE"=4, "SENSOR MODE"=5, "READOUT MODE"=6, "EXPOSURE TIME"=7, "CONTRAST GAIN"=8, "CONTRAST OFFSET"=9, "LIGHT MODE"=10, "SENSITIVITY"=11, "WHITE BALANCE"=12, "PHOTON IMAGING MODE"=13, "HIGH DYNAMIC RANGE MODE"=14, "TRIGGER SOURCE"=15, "TRIGGER ACTIVE"=16, "TRIGGER MODE"=17, "TRIGGER POLARITY"=18, "TRIGGER GLOBAL EXPOSURE"=19, "FIRST TRIGGER BEHAVIOR"=20, "TRIGGER TIMES"=21, "OUTPUT TRIGGER POLARITY"=22, "OUTPUT TRIGGER DELAY"=23, "OUTPUT TRIGGER PERIOD"=24, "TEMPERATURE"=25, "TEMPERATURE TARGET"=26, "SENSOR COOLER FAN"=27, "MECHANICAL SHUTTER"=28, "BACK FOCUS POSITION"=29, "FRAMEBUNDLE MODE"=30, "FRAMEBUNDLE NUMBER"=31, "LINEBUNDLE HEIGHT"=32, "TRIGGER CONNECTOR"=33, "IMAGE PIXEL TYPE"=34, "OUTPUT TRIGGER KIND"=35, "READOUT DIRECTION"=36, "CHANNEL SYNC"=37] ("Parameter")
                w372 = 1 items=["Snap", "Sequence"] ("Capture mode")
                n121 = event-data() -> ("NewVal"=w357:u16)  [unwired: 1 in, 2 out]
                n122 = call <userlib>:"tm_stopcapture_40.vi"("error in (no error)"=w364, "Handle in"=w365) -> ("error out"=w362:errorcluster, "Handle out"=w363:u32)  [unwired: 8 in]
                n123 = call <userlib>:"tm_unpreparecapture_40.vi"("error in (no error)"=w362, "Handle in"=w363) -> ("error out"=w360:errorcluster, "Handle out"=w358:u32)  [unwired: 8 in]
                n124 = call <userlib>:"tm_setparameter_40.vi"("error in (no error)"=w360, "Value in"=w357, "Parameter"=w359, "Handle in"=w358) -> ("error out"=w354:errorcluster, "Handle out"=w355:u32)  [unwired: 6 in]
                n125 = call <userlib>:"tm_getarea_40.vi"("error in (no error)"=w354, "Handle in"=w355) -> ("error out"=w352:errorcluster, "Sub Region"=w356:T5, "Handle out"=w353:u32)  [unwired: 7 in]
                n126 = Unbundle(w356) -> ("H Offset"=w343:cluster{"Value":i32, "Limits":T4}, "V Offset"=w342:cluster{"Value":i32, "Limits":T4}, "H Size"=w341:cluster{"Value":i32, "Limits":T4}, "V Size"=w340:cluster{"Value":i32, "Limits":T4})
                n127 = Unbundle By Name(w343) -> ("Value"=w351:i32, "Limits"=w350:T4)
                n128 = Unbundle By Name(w342) -> ("Value"=w349:i32, "Limits"=w348:T4)
                n129 = Unbundle By Name(w341) -> ("Value"=w347:i32, "Limits"=w346:T4)
                n130 = Unbundle By Name(w340) -> ("Value"=w345:i32, "Limits"=w344:T4)
                n131 = property on="H Offset" class="DigNum (strict)"("Value"=w351, "Data Range"=w350) -> ()  [unwired: 2 in, 2 out]
                n132 = property on="V Offset" class="DigNum (strict)"("Value"=w349, "Data Range"=w348) -> ()  [unwired: 2 in, 2 out]
                n133 = property on="H Width" class="DigNum (strict)"("Value"=w347, "Data Range"=w346) -> ()  [unwired: 2 in, 2 out]
                n134 = property on="V Width" class="DigNum (strict)"("Value"=w345, "Data Range"=w344) -> ()  [unwired: 2 in, 2 out]
                n135 = local write "SHO"(w351) -> ()
                n136 = local write "SVO"(w349) -> ()
                n137 = local write "SHW"(w347) -> ()
                n138 = local write "SVW"(w345) -> ()
                n139 = call <userlib>:"tm_preparecapture_40.vi"("error in (no error)"=w352, "Capture mode"=w372, "Handle in"=w353) -> ("error out"=w370:errorcluster, "Handle out"=w371:u32)  [unwired: 5 in, 2 out]
                n140 = call <userlib>:"tm_startcapture_40.vi"("error in (no error)"=w370, "Handle in"=w371) -> ("error out"=w369:errorcluster, "Handle out"=w368:u32)  [unwired: 8 in]
              }
              event "H Offset", "H Width", "V Offset", "V Width": Value Change {
                w386 = u32 4215968 items=["SENSOR MODE"=4212128, "READOUT SPEED"=4211872, "READOUT DIRECTION"=4211904, "TRIGGER GLOBAL EXPOSURE"=2049680, "TRIGGER DELAY"=1066480, "INTERNAL TRIGGER HANDLING"=1066496, "SENSOR TEMPERATURE"=2115232, "SENSOR COOLER STATUS"=2115280, "EXPOSURE TIME"=2049184, "DEFECT CORRECT MODE"=4670368, "HOT PIXEL CORRECT LEVEL"=4670400, "BINNING"=4215968, "TIMING READOUT TIME"=4223904, "INTERNAL FRAME RATE"=4225952, "INTERNAL FRAME INTERVAL"=4225968, "INTERNAL LINE SPEED"=4226000, "INTERNAL LINE INTERVAL"=4226016, "IMAGE WIDTH"=4343200, "IMAGE HEIGHT"=4343216, "IMAGE ROWBYTES"=4343232, "IMAGE FRAMEBYTES"=4343248, "IMAGE PIXEL TYPE"=4343296, "NUMBER OF OUTPUT TRIGGER CONNECTOR"=1852320, "OUTPUT TRIGGER SOURCE[0]"=1852576, "OUTPUT TRIGGER SOURCE[1]"=1852832, "OUTPUT TRIGGER SOURCE[2]"=1853088, "OUTPUT TRIGGER POLARITY[0]"=1852592, "OUTPUT TRIGGER POLARITY[1]"=1852848, "OUTPUT TRIGGER POLARITY[2]"=1853104, "OUTPUT TRIGGER ACTIVE[0]"=1852608, "OUTPUT TRIGGER ACTIVE[1]"=1852864, "OUTPUT TRIGGER ACTIVE[2]"=1853120, "OUTPUT TRIGGER DELAY[0]"=1852624, "OUTPUT TRIGGER DELAY[1]"=1852880, "OUTPUT TRIGGER DELAY[2]"=1853136, "OUTPUT TRIGGER PERIOD[0]"=1852640, "OUTPUT TRIGGER PERIOD[1]"=1852896, "OUTPUT TRIGGER PERIOD[2]"=1853152, "OUTPUT TRIGGER KIND[0]"=1852656, "OUTPUT TRIGGER KIND[1]"=1852912, "OUTPUT TRIGGER KIND[2]"=1853168, "OUTPUT TRIGGER BASE SENSOR[0]"=1852672, "OUTPUT TRIGGER BASE SENSOR[1]"=1852928, "OUTPUT TRIGGER BASE SENSOR[2]"=1853184, "OUTPUT TRIGGER PRE HSYNC COUNT"=1852704] ("Parameter")
                w418 = 1 items=["Snap", "Sequence"] ("Capture mode")
                n141 = event-data() -> ()  [unwired: 1 in, 4 out]
                n142 = call <userlib>:"tm_stopcapture_40.vi"("error in (no error)"=w409, "Handle in"=w410) -> ("error out"=w407:errorcluster, "Handle out"=w408:u32)  [unwired: 8 in]
                n143 = local read "H Offset"() -> (w383:i32)
                n144 = local read "H Width"() -> (w381:i32)
                n145 = local read "V Offset"() -> (w382:i32)
                n146 = local read "V Width"() -> (w380:i32)
                n147 = call <userlib>:"tm_unpreparecapture_40.vi"("error in (no error)"=w407, "Handle in"=w408) -> ("error out"=w387:errorcluster, "Handle out"=w388:u32)  [unwired: 8 in]
                n148 = call <userlib>:"tm_getparameter_40.vi"("error in (no error)"=w387, "Parameter"=w386, "Handle in"=w388) -> ("error out"=w384:errorcluster, "Value out"=w375:dbl, "Handle out"=w385:u32)  [unwired: 6 in]
                n149 = To Long Integer(number=w375) -> (32bit integer=w374:i32)
                n150 = Multiply(x=w380, y=w374) -> (x*y=w376:i32)
                n151 = Multiply(x=w381, y=w374) -> (x*y=w377:i32)
                n152 = Multiply(x=w382, y=w374) -> (x*y=w378:i32)
                n153 = Multiply(x=w383, y=w374) -> (x*y=w379:i32)
                n154 = Bundle(w379, w378, w377, w376) -> (w411:cluster{i32, i32, i32, i32})  [unwired: 1 in]
                n155 = call <userlib>:"tm_setarea_40.vi"("error in (no error)"=w384, "Sub Region"=w411, "Handle in"=w385) -> ("error out"=w404:errorcluster, "Handle out"=w405:u32)  [unwired: 7 in]
                n156 = call <userlib>:"tm_getarea_40.vi"("error in (no error)"=w404, "Handle in"=w405) -> ("error out"=w402:errorcluster, "Sub Region"=w394:T5, "Handle out"=w403:u32)  [unwired: 7 in]
                n157 = Unbundle(w394) -> ("H Offset"=w401:cluster{"Value":i32, "Limits":T4}, "V Offset"=w400:cluster{"Value":i32, "Limits":T4}, "H Size"=w399:cluster{"Value":i32, "Limits":T4}, "V Size"=w398:cluster{"Value":i32, "Limits":T4})
                n158 = Unbundle By Name(w401) -> ("Value"=w397:i32, "Limits"=w396:T4)
                n159 = Unbundle By Name(w400) -> ("Value"=w395:i32, "Limits"=w390:T4)
                n160 = Unbundle By Name(w399) -> ("Value"=w391:i32, "Limits"=w389:T4)
                n161 = Unbundle By Name(w398) -> ("Value"=w393:i32, "Limits"=w392:T4)
                n162 = property on="H Offset" class="DigNum (strict)"("Value"=w397, "Data Range"=w396) -> ()  [unwired: 2 in, 2 out]
                n163 = property on="V Offset" class="DigNum (strict)"("Value"=w395, "Data Range"=w390) -> ()  [unwired: 2 in, 2 out]
                n164 = property on="H Width" class="DigNum (strict)"("Value"=w391, "Data Range"=w389) -> ()  [unwired: 2 in, 2 out]
                n165 = property on="V Width" class="DigNum (strict)"("Value"=w393, "Data Range"=w392) -> ()  [unwired: 2 in, 2 out]
                n166 = call <userlib>:"tm_preparecapture_40.vi"("error in (no error)"=w402, "Capture mode"=w418, "Handle in"=w403) -> ("error out"=w416:errorcluster, "Handle out"=w417:u32)  [unwired: 5 in, 2 out]
                n167 = local write "SHO"(w397) -> ()
                n168 = local write "SVO"(w395) -> ()
                n169 = local write "SHW"(w391) -> ()
                n170 = local write "SVW"(w393) -> ()
                n171 = call <userlib>:"tm_startcapture_40.vi"("error in (no error)"=w416, "Handle in"=w417) -> ("error out"=w415:errorcluster, "Handle out"=w414:u32)  [unwired: 8 in]
              }
            }
            n172 = Unbundle By Name(w236) -> ("status"=w248:bool)
            n173 = Or(x=w248, y="stop") -> (x .or. y?=w247:bool)
          }
          n174 = call <userlib>:"tm_stopcapture_40.vi"("error in (no error)"=w218, "Handle in"=w219) -> ("error out"=w215:errorcluster, "Handle out"=w216:u32)  [unwired: 8 in]
          n175 = call <userlib>:"tm_unpreparecapture_40.vi"("error in (no error)"=w215, "Handle in"=w216) -> ("error out"=w214:errorcluster, "Handle out"=w217:u32)  [unwired: 8 in]
          n176 = call <userlib>:"tm_closecamera_40.vi"("error in (no error)"=w214, "Handle in"=w217) -> ("error out"=w228:errorcluster)  [unwired: 9 in]
          n177 = call <userlib>:"tm_deinitialize_40.vi"("error in (no error)"=w228) -> ("error out"=w227:errorcluster)  [unwired: 10 in]
        }
      }
      "error out" <- w55
      n178 = while {
        tunnel: w69 -> [w699]
        tunnel: [w698] -> w67
        tunnel: w68 -> [w697]
        tunnel: [w696] -> w66
        tunnel: w65 -> [w694]
        shift-right: [w638] -> _
        shift-left: _ -> [w637]
        stop <- FALSE stop-if-true
        (unwired) 200000.0 ("y")
        n179 = Tick Count (ms)() -> (millisecond timer value=w693:u32)
        n180 = Subtract(x=w693, y=w694) -> (x-y=w688:u32)
        n181 = Divide(x="Threshold1", y="ratiocontrol") -> (x/y=w681:dbl)
        n182 = Divide(x="Threshold2", y="ratiocontrol") -> (x/y=w680:dbl)
        n183 = Multiply(x="determine ratio (xx.xx)", y=100.0) -> (x*y=w661:dbl)
        n184 = Multiply(x="Droplet width [ms]", y=0.001) -> (x*y=w663:dbl)
        n185 = Multiply(x=0.001, y=w688) -> (x*y=w655:dbl)
        "LabView Timer (sec)" <- w655
        n186 = Quotient & Remainder(x=w688, y=u32 1) -> (x-y*floor(x/y)=w690:u32)  [unwired: 1 out]
        n187 = Multiply(x=w663, y=w637) -> (x*y=w662:dbl)
        n188 = To Unsigned Quad Integer(1:w662) -> (0:w676:u64)
        n189 = xnode "Read/Write Control"("FPGA VI Reference In"=w699, "error in"=w697, "Threshold1"=w681, "Threshold2"=w680, "Time compensation [clock]"=w676, "FPGA initializer"="FPGA initializer", "determine ratio"=w661) -> ("FPGA VI Reference Out"=w698:refnum<k20>, "error out"=w696:errorcluster, "Sort"=w679:bool, "Unfiltered  Signal1"=w658:i16, "Filtered Signal1"=w646:i16, "Unfiltered  Signal2"=w682:i16, "Filtered Signal2"=w657:i16, "t0 (sample)"=→"t0 (sample)":u64, "t1 (sample)"=→"t1 (sample)":u64, "Droplet counter"=→"Droplet counter":u64, "Sorted droplet counter"=→"Sorted droplet counter":u64, "loop counter"=w667:u64, "Droplet lock on"=→"Droplet lock on":bool, "PMT1 sum"=w640:u64, "PMT2 sum"=w639:u64, "sample diff"=→"sample diff":u64, "Loop length (uSec)"=w666:u32)  [unwired: 1 out]
        "Unfiltered Signal 1" <- w658
        "Filtered Signal 2" <- w657
        "Unfiltered Signal 2" <- w682
        "PMT1 sum" <- w640
        "PMT2 sum" <- w639
        "FPGA loop counter" <- w667
        "Sort" <- w679
        "Filtered Signal 1" <- w646
        "PMT1 sum" <- w640
        "PMT2 sum" <- w639
        n190 = case shown="0" w690 {
          tunnel: w682 -> [_ w715]
          tunnel: w657 -> [_ w714]
          tunnel: w646 -> [_ w713]
          tunnel: w658 -> [_ w712]
          tunnel: w680 -> [_ w710]
          tunnel: w681 -> [_ w709]
          tunnel: w679 -> [_ w707]
          tunnel: w655 -> [_ w705]
          tunnel: "ratiocontrol" -> [_ w703]
          frame Default {
          }
          frame 0 {
            n191 = Number To Fractional String(number=w705) -> (F-format string=w704:string)  [unwired: 3 in]
            n192 = Format Into String(w709) -> (resulting string=w717:string)  [unwired: 3 in, 1 out]
            n193 = Multiply(x=w712, y=w703) -> (x*y=w725:dbl)
            n194 = Format Into String(w725) -> (resulting string=w716:string)  [unwired: 3 in, 1 out]
            n195 = Multiply(x=w713, y=w703) -> (x*y=w726:dbl)
            n196 = Format Into String(w710) -> (resulting string=w719:string)  [unwired: 3 in, 1 out]
            n197 = Format Into String(w726) -> (resulting string=w718:string)  [unwired: 3 in, 1 out]
            n198 = Format Into String(w707) -> (resulting string=w706:string)  [unwired: 3 in, 1 out]
            n199 = Multiply(x=w715, y=w703) -> (x*y=w727:dbl)
            n200 = Format Into String(w727) -> (resulting string=w720:string)  [unwired: 3 in, 1 out]
            n201 = Multiply(x=w714, y=w703) -> (x*y=w728:dbl)
            n202 = Format Into String(w728) -> (resulting string=w721:string)  [unwired: 3 in, 1 out]
            n203 = Build Array(w717, w716, w718, w706, w704, "" ("element"), w719, w720, w721, w706, w704) -> (w723:string[])
            n204 = Array To Spreadsheet String(array=w723, 3:"%s" ("format string")) -> (spreadsheet string=w722:string)  [unwired: 1 in]
            n205 = local read "Data File Ptr"() -> (w724:refnum<file>)
            n206 = Write to Text File(file (use dialog)=w724, text=w722) -> ()  [unwired: 2 in, 3 out]
          }
        }
        n207 = To Double Precision Float(number=w640) -> (double precision float=w645:dbl)
        n208 = To Double Precision Float(number=w639) -> (double precision float=w644:dbl)
        n209 = Divide(x=w645, y=w644) -> (x/y=w641:dbl)
        n210 = Not A Number/Path/Refnum?(number/path/refnum=w641) -> (NaN/Path/Refnum?=w643:bool)
        n211 = case shown="False" w643 {
          tunnel: [w700 0.0] -> w642
          tunnel: w641 -> [w700 _]
          frame False {
          }
          frame True {
          }
        }
        "PMT1/PMT2" <- w642
        "PMT1/PMT2 (graph)" <- w642
        n212 = Multiply(x="ratiocontrol", y=w658) -> (x*y=→"Unfiltered Signal1":dbl)
        n213 = Divide(x=w666, y=1000000.0 ("x")) -> (x/y=w664:dbl)
        n214 = call "Tick Count"() -> ("Tick Count(uSec)"=w648:u32)
        n215 = Divide(x=1.0, y=w664) -> (x/y=w638:dbl)
        "FPGA freq" <- w638
        n216 = local read "FPGA initializer"() -> (w668:bool)
        n217 = Divide(x=w667, y=w638) -> (x/y=→"FPGA timer (sec)":dbl)
        n218 = feedback #1() -> (w647:u32)  [unwired: 1 in]
        n219 = feedback-in #1(w648) -> ()
        n220 = Multiply(x="ratiocontrol", y=w646) -> (x*y=→"Filtered Signal1":dbl)
        n221 = Subtract(x=w648, y=w647) -> (x-y=w649:u32)
        n222 = case shown="True" w668 {
          frame False {
          }
          frame True {
            n223 = local write "FPGA initializer"(FALSE ("FPGA initializer")) -> ()
          }
        }
        n224 = Multiply(x="ratiocontrol", y=w682) -> (x*y=→"Unfiltered Signal2":dbl)
        n225 = Divide(x=w649, y=1000000.0 ("x")) -> (x/y=w652:dbl)
        n226 = Multiply(x="ratiocontrol", y=w657) -> (x*y=→"Filtered Signal2":dbl)
        n227 = Divide(x=1.0, y=w652) -> (x/y=→"LabView freq":dbl)
      }
      n228 = while {
        shift-right: [w420] -> w57
        shift-left: w60 -> [w508]
        shift-right: [w423] -> w61
        shift-left: w59 -> [w507]
        shift-right: [w421] -> _
        shift-left: _ -> [w505]
        stop <- "Arduino \nshut down" continue-if-true
        n229 = case shown="True" "Initializer" {
          tunnel: w508 -> [w625 w635]
          tunnel: w507 -> [w626 w634]
          tunnel: [w625 w631] -> w504
          tunnel: [w626 w630] -> w503
          tunnel: w505 -> [w627 w629]
          tunnel: [w627 w629] -> w502
          frame False {
          }
          frame True {
            n230 = local write "Initializer"(FALSE ("send")) -> ()
            n231 = Wait (ms)(milliseconds to wait=u32 100) -> ()  [unwired: 1 out]
            n232 = VISA Write(VISA resource name=w635, write buffer="LV_INIT", error in (no error)=w634) -> (VISA resource name out=w631:refnum<visa-resource-name>, error out=w630:errorcluster)  [unwired: 1 out]
          }
        }
        n233 = Divide(x="PMT1 senstivity input", y=5.0) -> (x/y=w474:dbl)
        n234 = Multiply(x=w474, y=128.0) -> (x*y=w476:dbl)
        n235 = Subtract(x=w476, y=1.0) -> (x-y=w471:dbl)
        n236 = Round To Nearest(number=w471) -> (nearest integer value=w480:dbl)
        n237 = Format Into String(w480) -> (resulting string=w479:string)  [unwired: 3 in, 1 out]
        n238 = Concatenate Strings("POT1 " ("string"), w479) -> (w477:string)
        n239 = Divide(x="PMT2 senstivity input", y=5.0) -> (x/y=w466:dbl)
        n240 = case shown="False" "PMT1 senstivity" {
          tunnel: w504 -> [w615 w624]
          tunnel: w503 -> [w614 w623]
          tunnel: [w615 w620] -> w501
          tunnel: [w614 w619] -> w500
          tunnel: w502 -> [w616 w618]
          tunnel: [w616 w618] -> w499
          tunnel: w477 -> [_ w617]
          frame False {
          }
          frame True {
            n241 = VISA Write(VISA resource name=w624, write buffer=w617, error in (no error)=w623) -> (VISA resource name out=w620:refnum<visa-resource-name>, error out=w619:errorcluster)  [unwired: 1 out]
            n242 = local write "PMT1 senstivity"(FALSE ("send")) -> ()
            n243 = Wait (ms)(milliseconds to wait=u32 100) -> ()  [unwired: 1 out]
          }
        }
        n244 = Multiply(x=w466, y=128.0) -> (x*y=w464:dbl)
        n245 = Subtract(x=w464, y=1.0) -> (x-y=w468:dbl)
        n246 = Round To Nearest(number=w468) -> (nearest integer value=w461:dbl)
        n247 = Format Into String(w461) -> (resulting string=w462:string)  [unwired: 3 in, 1 out]
        n248 = Concatenate Strings("POT2 " ("string"), w462) -> (w459:string)
        n249 = case shown="False" "PMT2 senstivity" {
          tunnel: w501 -> [w603 w613]
          tunnel: w500 -> [w604 w612]
          tunnel: [w603 w609] -> w488
          tunnel: [w604 w608] -> w487
          tunnel: w499 -> [w605 w607]
          tunnel: [w605 w607] -> w489
          tunnel: w459 -> [_ w606]
          frame False {
          }
          frame True {
            n250 = VISA Write(VISA resource name=w613, write buffer=w606, error in (no error)=w612) -> (VISA resource name out=w609:refnum<visa-resource-name>, error out=w608:errorcluster)  [unwired: 1 out]
            n251 = local write "PMT2 senstivity"(FALSE ("send")) -> ()
            n252 = Wait (ms)(milliseconds to wait=u32 100) -> ()  [unwired: 1 out]
          }
        }
        n253 = Divide(x="Func amp input", y=5.0) -> (x/y=w453:dbl)
        n254 = Multiply(x=w453, y=128.0) -> (x*y=w455:dbl)
        n255 = Subtract(x=w455, y=1.0) -> (x-y=w451:dbl)
        n256 = Round To Nearest(number=w451) -> (nearest integer value=w457:dbl)
        n257 = Format Into String(w457) -> (resulting string=w456:string)  [unwired: 3 in, 1 out]
        n258 = Concatenate Strings("POT_HV AMP " ("string"), w456) -> (w449:string)
        n259 = case shown="False" "Func amp" {
          tunnel: w488 -> [w594 w602]
          tunnel: w487 -> [w592 w601]
          tunnel: [w594 w598] -> w498
          tunnel: [w592 w597] -> w497
          tunnel: w489 -> [w593 w596]
          tunnel: [w593 w596] -> w496
          tunnel: w449 -> [_ w595]
          frame False {
          }
          frame True {
            n260 = VISA Write(VISA resource name=w602, write buffer=w595, error in (no error)=w601) -> (VISA resource name out=w598:refnum<visa-resource-name>, error out=w597:errorcluster)  [unwired: 1 out]
            n261 = local write "Func amp"(FALSE ("send")) -> ()
            n262 = Wait (ms)(milliseconds to wait=u32 100) -> ()  [unwired: 1 out]
          }
        }
        n263 = Format Into String("Func freq input") -> (resulting string=w448:string)  [unwired: 3 in, 1 out]
        n264 = Concatenate Strings("POT_HV FRQ " ("string"), w448) -> (w445:string)
        n265 = case shown="False" "Func Freq" {
          tunnel: w498 -> [w582 w591]
          tunnel: w497 -> [w581 w590]
          tunnel: [w582 w587] -> w490
          tunnel: [w581 w586] -> w491
          tunnel: w496 -> [w583 w585]
          tunnel: [w583 w585] -> w495
          tunnel: w445 -> [_ w584]
          frame False {
          }
          frame True {
            n266 = VISA Write(VISA resource name=w591, write buffer=w584, error in (no error)=w590) -> (VISA resource name out=w587:refnum<visa-resource-name>, error out=w586:errorcluster)  [unwired: 1 out]
            n267 = local write "Func Freq"(FALSE ("send")) -> ()
            n268 = Wait (ms)(milliseconds to wait=u32 100) -> ()  [unwired: 1 out]
          }
        }
        n269 = Multiply(x="Func on Time input", y=1000.0) -> (x*y=w435:dbl)
        n270 = Format Into String(w435) -> (resulting string=w444:string)  [unwired: 3 in, 1 out]
        n271 = Concatenate Strings("POT_HV ONT " ("string"), w444) -> (w443:string)
        n272 = case shown="False" "Func On time" {
          tunnel: w491 -> [w570 w580]
          tunnel: [w571 w577] -> w493
          tunnel: [w570 w576] -> w492
          tunnel: w495 -> [w572 w575]
          tunnel: [w572 w575] -> w494
          tunnel: w490 -> [w571 w574]
          tunnel: w443 -> [_ w573]
          frame False {
          }
          frame True {
            n273 = VISA Write(VISA resource name=w574, write buffer=w573, error in (no error)=w580) -> (VISA resource name out=w577:refnum<visa-resource-name>, error out=w576:errorcluster)  [unwired: 1 out]
            n274 = local write "Func On time"(FALSE ("send")) -> ()
            n275 = Wait (ms)(milliseconds to wait=u32 100) -> ()  [unwired: 1 out]
          }
        }
        n276 = Multiply(x="Func delay input", y=1000.0) -> (x*y=w433:dbl)
        n277 = Format Into String(w433) -> (resulting string=w442:string)  [unwired: 3 in, 1 out]
        n278 = Concatenate Strings("POT_HV DLY " ("string"), w442) -> (w441:string)
        n279 = case shown="True" "Func Delay" {
          tunnel: w493 -> [w561 w569]
          tunnel: w492 -> [w560 w568]
          tunnel: [w561 w565] -> w425
          tunnel: [w560 w564] -> w424
          tunnel: w494 -> [w559 w563]
          tunnel: [w559 w563] -> w422
          tunnel: w441 -> [_ w562]
          frame False {
          }
          frame True {
            n280 = VISA Write(VISA resource name=w569, write buffer=w562, error in (no error)=w568) -> (VISA resource name out=w565:refnum<visa-resource-name>, error out=w564:errorcluster)  [unwired: 1 out]
            n281 = local write "Func Delay"(FALSE ("send")) -> ()
            n282 = Wait (ms)(milliseconds to wait=u32 100) -> ()  [unwired: 1 out]
          }
        }
        n283 = feedback #2(FALSE ("Motor Start/Stop")) -> (w429:bool)
        n284 = feedback-in #2("Merger on") -> ()
        n285 = Build Array("Merger on", w429) -> (w428:bool[])
        n286 = Boolean Array To Number(Boolean array=w428) -> (number=w431:u32)
        n287 = case shown="1" w431 {
          tunnel: "MERGE " ("string") -> [_ w524 w544]
          tunnel: w422 -> [_ w519 w542]
          tunnel: [w514 w520 w541] -> w420
          tunnel: [w510 w519 w542] -> w421
          tunnel: [w513 w521 w543] -> w423
          tunnel: w424 -> [w512 w522 w540]
          tunnel: w425 -> [w511 w523 w539]
          frame 0, Default {
            n288 = Wait (ms)(milliseconds to wait=u32 100) -> ()  [unwired: 1 out]
            n289 = property class="Instr"(reference=w511, error in=w512) -> (reference out=w517:refnum<visa-resource-name>, error out=w515:errorcluster, "Bytes at Port"=w516:u32)
            n290 = VISA Read(VISA resource name=w517, byte count=w516, error in (no error)=w515) -> (VISA resource name out=w514:refnum<visa-resource-name>, read buffer=w510:string, error out=w513:errorcluster)  [unwired: 1 out]
            "Serial debugger" <- w510
          }
          frame 1 {
            n291 = Concatenate Strings(w524, "ON " ("string")) -> (w527:string)
            n292 = flat-sequence {
              tunnel: w527 -> [w534]
              tunnel: w523 -> [w533]
              tunnel: w522 -> [w532]
              tunnel: [w531] -> w526
              tunnel: [w530] -> w525
              tunnel: w526 -> [w538]
              tunnel: w525 -> [w537]
              tunnel: [w536] -> w520
              tunnel: [w535] -> w521
              frame #0 {
                n293 = VISA Write(VISA resource name=w533, write buffer=w534, error in (no error)=w532) -> (VISA resource name out=w531:refnum<visa-resource-name>, error out=w530:errorcluster)  [unwired: 1 out]
                n294 = Wait Until Next ms Multiple(millisecond multiple=u32 100) -> ()  [unwired: 1 out]
              }
              frame #1 {
                n295 = VISA Clear(VISA resource name=w538, error in (no error)=w537) -> (VISA resource name out=w536:refnum<visa-resource-name>, error out=w535:errorcluster)
              }
            }
          }
          frame 2 {
            n296 = Concatenate Strings(w544, "OFF " ("string")) -> (w547:string)
            n297 = flat-sequence {
              tunnel: w547 -> [w554]
              tunnel: w539 -> [w551]
              tunnel: w540 -> [w550]
              tunnel: [w553] -> w546
              tunnel: [w552] -> w545
              tunnel: [w558] -> w543
              tunnel: [w555] -> w541
              tunnel: w546 -> [w557]
              tunnel: w545 -> [w556]
              frame #0 {
                n298 = VISA Write(VISA resource name=w551, write buffer=w554, error in (no error)=w550) -> (VISA resource name out=w553:refnum<visa-resource-name>, error out=w552:errorcluster)  [unwired: 1 out]
                n299 = Wait Until Next ms Multiple(millisecond multiple=u32 100) -> ()  [unwired: 1 out]
              }
              frame #1 {
                n300 = VISA Clear(VISA resource name=w557, error in (no error)=w556) -> (VISA resource name out=w555:refnum<visa-resource-name>, error out=w558:errorcluster)
              }
            }
          }
        }
      }
      n301 = xnode "Close FPGA VI Reference"("FPGA VI Reference In"=w67, "error in"=w66) -> ()  [unwired: 1 out]
      n302 = call <instrlib>:"Stop Pump.vi"("error in (no error)"=w47, "VISA resource name"=w48) -> ("error out"=w51:errorcluster, "VISA resource name out"=w50:refnum<visa-resource-name>)  [unwired: 8 in]
      n303 = call <instrlib>:"Close.vi"("error in (no error)"=w51, "VISA resource name"=w50) -> ("error out"=w49:errorcluster)  [unwired: 9 in]
      n304 = call <vilib>:"Simple Error Handler.vi"("error in (no error)"=w49) -> ()  [unwired: 4 in, 5 out]
      n305 = VISA Close(VISA resource name=w57, error in (no error)=w61) -> (error out=w62:errorcluster)
      n306 = call <vilib>:"Simple Error Handler.vi"("error in (no error)"=w62) -> ()  [unwired: 4 in, 5 out]
    }
    frame #2 {
      n307 = local read "Data File Ptr"() -> (w729:refnum<file>)
      n308 = Close File(refnum=w729) -> ()  [unwired: 1 in, 2 out]
    }
  }
